vi "testCreation1024.vi"(8 "error in (no error)":errorcluster, 11 "TestCase in":refnum<class "Creation.lvclass">) -> (0 "error out":errorcluster, 3 "TestCase out":refnum<class "Creation.lvclass">)   [LabVIEW 2017, in "Deterministic Error Tests.lvlib" / "Creation.lvclass"]
uses:
  Creation.lvclass
  Source/VIs/VIs for Poly/Create Error Cluster (1024B).vi
  Source/Deterministic Error Builder.lvlib
  <vilib>/addons/_JKI Toolkits/VI Tester/TestCase.llb/TestCase.lvclass
  C:/Program Files (x86)/National Instruments/LabVIEW 2017/vi.lib/addons/_JKI Toolkits/VI Tester/TestCase.llb/TestCase.lvclass
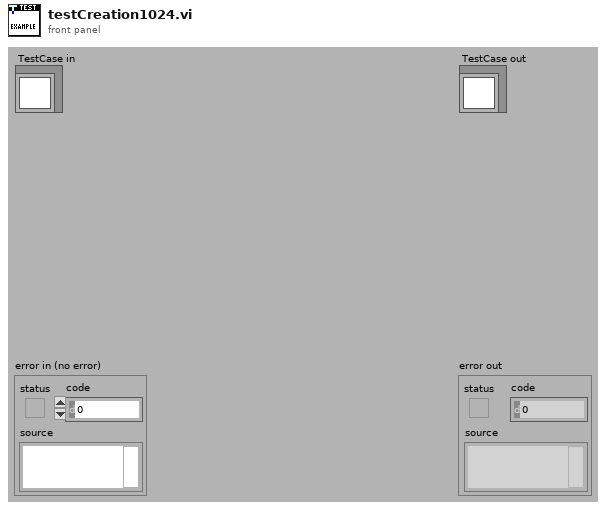
[diagram p1: front panel]
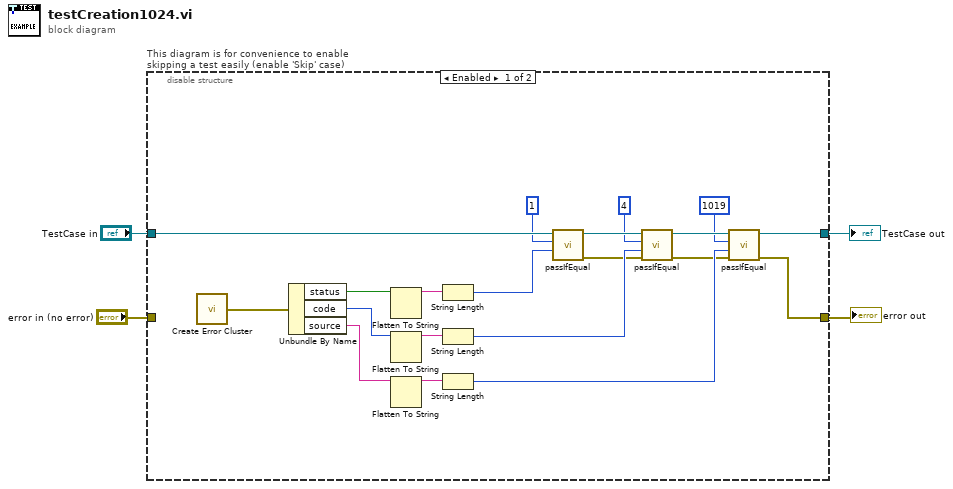
[diagram p0: block diagram]
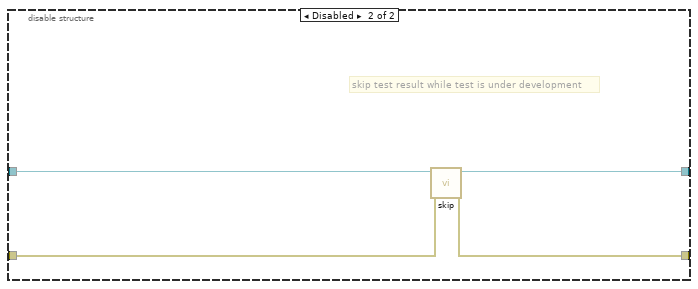
[diagram p2: hidden frame]
diagram:
  n1 = disable-structure "This diagram is for convenience to enable skipping a test easily (enable 'Skip' case)" shown="Enabled" {
    disable-tunnel: "TestCase in" -> [w24 w28]
    disable-tunnel: [w7 w26] -> w2
    disable-tunnel: [w6 w27] -> w1
    disable-tunnel: "error in (no error)" -> [_ w25]
    frame Enabled {
      n2 = call-poly "Create Error Cluster.vi"() -> ("error out"=w23:errorcluster)  [unwired: 1 in]
      n3 = Unbundle By Name(w23) -> ("status"=w22:bool, "code"=w21:i32, "source"=w20:string)
      n4 = Flatten To String(anything=w22) -> (data string=w19:string)  [unwired: 3 in, 2 out]
      n5 = Flatten To String(anything=w21) -> (data string=w18:string)  [unwired: 3 in, 2 out]
      n6 = Flatten To String(anything=w20) -> (data string=w17:string)  [unwired: 3 in, 2 out]
      n7 = String Length(string=w19) -> (length=w5:i32)
      n8 = String Length(string=w18) -> (length=w11:i32)
      n9 = String Length(string=w17) -> (length=w9:i32)
      n10 = call-dynamic "passIfEqual.vi"("y"=w5, "x"=1 ("length"), "TestCase in"=w24) -> ("error out"=w10:errorcluster, "TestCase out"=w15:refnum<class "Creation.lvclass">)  [unwired: 7 in]
      n11 = call-dynamic "passIfEqual.vi"("error in (no error)"=w10, "y"=w11, "x"=4 ("length"), "TestCase in"=w15) -> ("error out"=w8:errorcluster, "TestCase out"=w14:refnum<class "Creation.lvclass">)  [unwired: 6 in]
      n12 = call-dynamic "passIfEqual.vi"("error in (no error)"=w8, "y"=w9, "x"=1019 ("length"), "TestCase in"=w14) -> ("error out"=w6:errorcluster, "TestCase out"=w7:refnum<class "Creation.lvclass">)  [unwired: 6 in]
    }
    frame Disabled {
      # "skip test result while test is under development"
      n13 = call <vilib>:"skip.vi"("error in (no error)"=w25, "TestCase in"=w28) -> ("error out"=w27:errorcluster, "TestCase out"=w26:refnum<class "Creation.lvclass">)  [unwired: 8 in]
    }
  }
  "error out" <- w1
  "TestCase out" <- w2
